vi "Configure Power Factor High Limit.vi"(0 "VISA resource name":refnum<visa-resource-name>, 5 "Power Factor High Limit (0)":dbl min=0.0 max=1.0 format="%.3f", 11 "error in (no error)":errorcluster) -> (4 "VISA resource name out":refnum<visa-resource-name>, 15 "error out":errorcluster)   [LabVIEW 2016, in "APT 300XAC Series.lvlib"]
doc: "Sets <B>power factor high Limit</B> of the power source instrument.\n\n<B>Range</B> : 0.000~1.000\n\nThe Power Factor High-Limit setting configures a maximum power factor threshold or ceiling level. When this level is reached a test failure will occur."
uses:
  APT 300XAC Series.lvlib
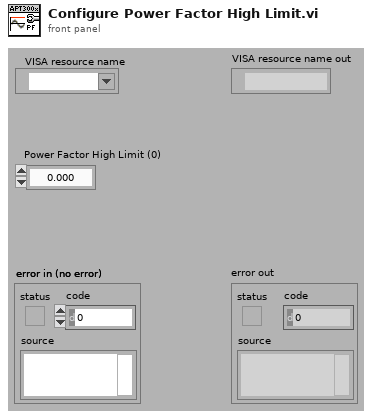
[diagram p1: front panel]
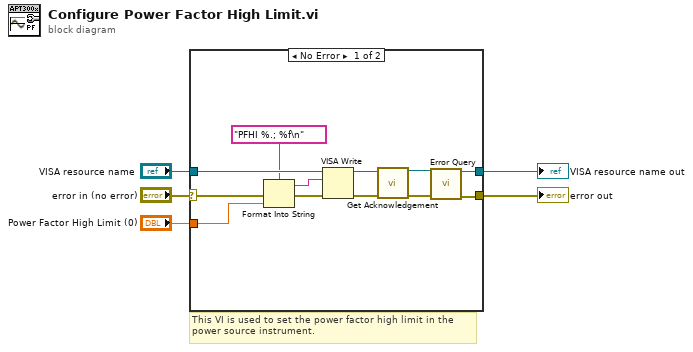
[diagram p0: block diagram]
diagram:
  # "This VI is used to set the power factor high limit in the\npower source instrument."
  n1 = case shown="No Error" "error in (no error)" {
    selector: "error in (no error)" -> [w11 w19]
    tunnel: [w12 w19] -> w5
    tunnel: [w13 w18] -> w4
    tunnel: "VISA resource name" -> [w17 w18]
    tunnel: "Power Factor High Limit (0)" -> [w16 _]
    frame No Error {
      n2 = Format Into String(format string="PFHI %.; %f\n" ("Command"), error in=w11, w16) -> (resulting string=w15:string, error out=w10:errorcluster)  [unwired: 1 in]
      n3 = VISA Write(VISA resource name=w17, write buffer=w15, error in (no error)=w10) -> (VISA resource name out=w9:refnum<visa-resource-name>, error out=w8:errorcluster)  [unwired: 1 out]
      n4 = call "Get Acknowledgement.vi"("VISA resource name"=w9, "error in (no error)"=w8) -> ("VISA resource name out"=w6:refnum<visa-resource-name>, "error out"=w7:errorcluster)  [unwired: 12 in]
      n5 = call "Error Query.vi"("VISA resource name"=w6, "error in (no error)"=w7) -> ("VISA resource name out"=w13:refnum<visa-resource-name>, "error out"=w12:errorcluster)  [unwired: 10 in, 2 out]
    }
    frame Error {
    }
  }
  "error out" <- w5
  "VISA resource name out" <- w4
